vi "OEE_SCREEN_2_worst_ok_count_into_cluster.vi"(6 "SCREEN_2":T1={"header_part_no"="-", "header_customer"="-", "performance_percentage"="-", "performance_target"="-", "performance_actual"="-", "performance_header"="PERFORMANCE", "performance_header_target"="TARGET", "performance_header_actual"="ACTUAL"}, 11 "SCREEN_1":T2={"header_date"="-", "header_time"="-", "header_takt"="-", "header_shift"="-", "OP10_actual"="-", "OP10_rejects"="-", "OP10_quality_yeild"="-", "OP10_pace"="-", "OP20_actual"="-", "OP20_rejects"="-", "OP20_quality_yeild"="-", "OP20_pace"="-", "OP30_actual"="-", "OP30_rejects"="-", "OP30_quality_yeild"="-", "OP30_pace"="-", "OP40_actual"="-", "OP40_rejects"="-", "OP40_quality_yeild"="-", "OP40_pace"="-", "OP50_actual"="-", "OP50_rejects"="-", "OP50_quality_yeild"="-", "OP50_pace"="-", "OP60_actual"="-", "OP60_rejects"="-", "OP60_quality_yeild"="-", "OP60_pace"="-", "OP70_actual"="-", "OP70_rejects"="-", "OP70_quality_yeild"="-", "OP70_pace"="-", "OP80_actual"="-", "OP80_rejects"="-", "OP80_quality_yeild"="-", "OP80_pace"="-", "OP90_actual"="-", "OP90_rejects"="-", "OP90_quality_yeild"="-", "OP90_pace"="-", "OP100_actual"="-", "OP100_rejects"="-", "OP100_quality_yeild"="-", "OP100_pace"="-", "OP110_actual"="-", "OP110_rejects"="-", "OP110_quality_yeild"="-", "OP110_pace"="-", "OP120_actual"="-", "OP120_rejects"="-", "OP120_quality_yeild"="-", "OP120_pace"="-", "OP130_actual"="-", "OP130_rejects"="-", "OP130_quality_yeild"="-", "OP130_pace"="-", "OP10_header"="OP10", "OP20_header"="OP20", "OP30_header"="OP30", "OP40_header"="OP40", "OP50_header"="OP50", "OP60_header"="OP60", "OP70_header"="OP70", "OP80_header"="OP80", "OP90_header"="OP90", "OP100_header"="OP100", "OP110_header"="OP110", "OP120_header"="OP120", "OP130_header"="OP130", "additional_info"="", "bottleneck_OP"="-", "bottleneck_header"="LINE BOTTLENECK"}) -> (4 "SCREEN_2":T1={"header_part_no"="-", "header_customer"="-", "performance_percentage"="-", "performance_target"="-", "performance_actual"="-", "performance_header"="PERFORMANCE", "performance_header_target"="TARGET", "performance_header_actual"="ACTUAL"})   [LabVIEW 2019]
uses:
  <userlib>/_OpenG.lib/array/array.llb/Sort 1D Array (I32)__ogtk.vi
  <userlib>/_OpenG.lib/array/array.llb/Reorder 2D Array2 (String)__ogtk.vi
  SCREEN_1/typedef/SCREEN_1.ctl
  typedef/SCREEN_2.ctl
panel:
  # "Performance Data Output Board #2"
  # "Performance Data Output Board #2"
  # "PERFORMANCE DATA OUTPUT BOARD #1"
  # "OP"
  # "Actual"
  # "Rejects"
  # "%FTTH"
  # "Pace"
  # "OP"
  # "Actual"
  # "Rejects"
  # "%FTTH"
  # "Pace"
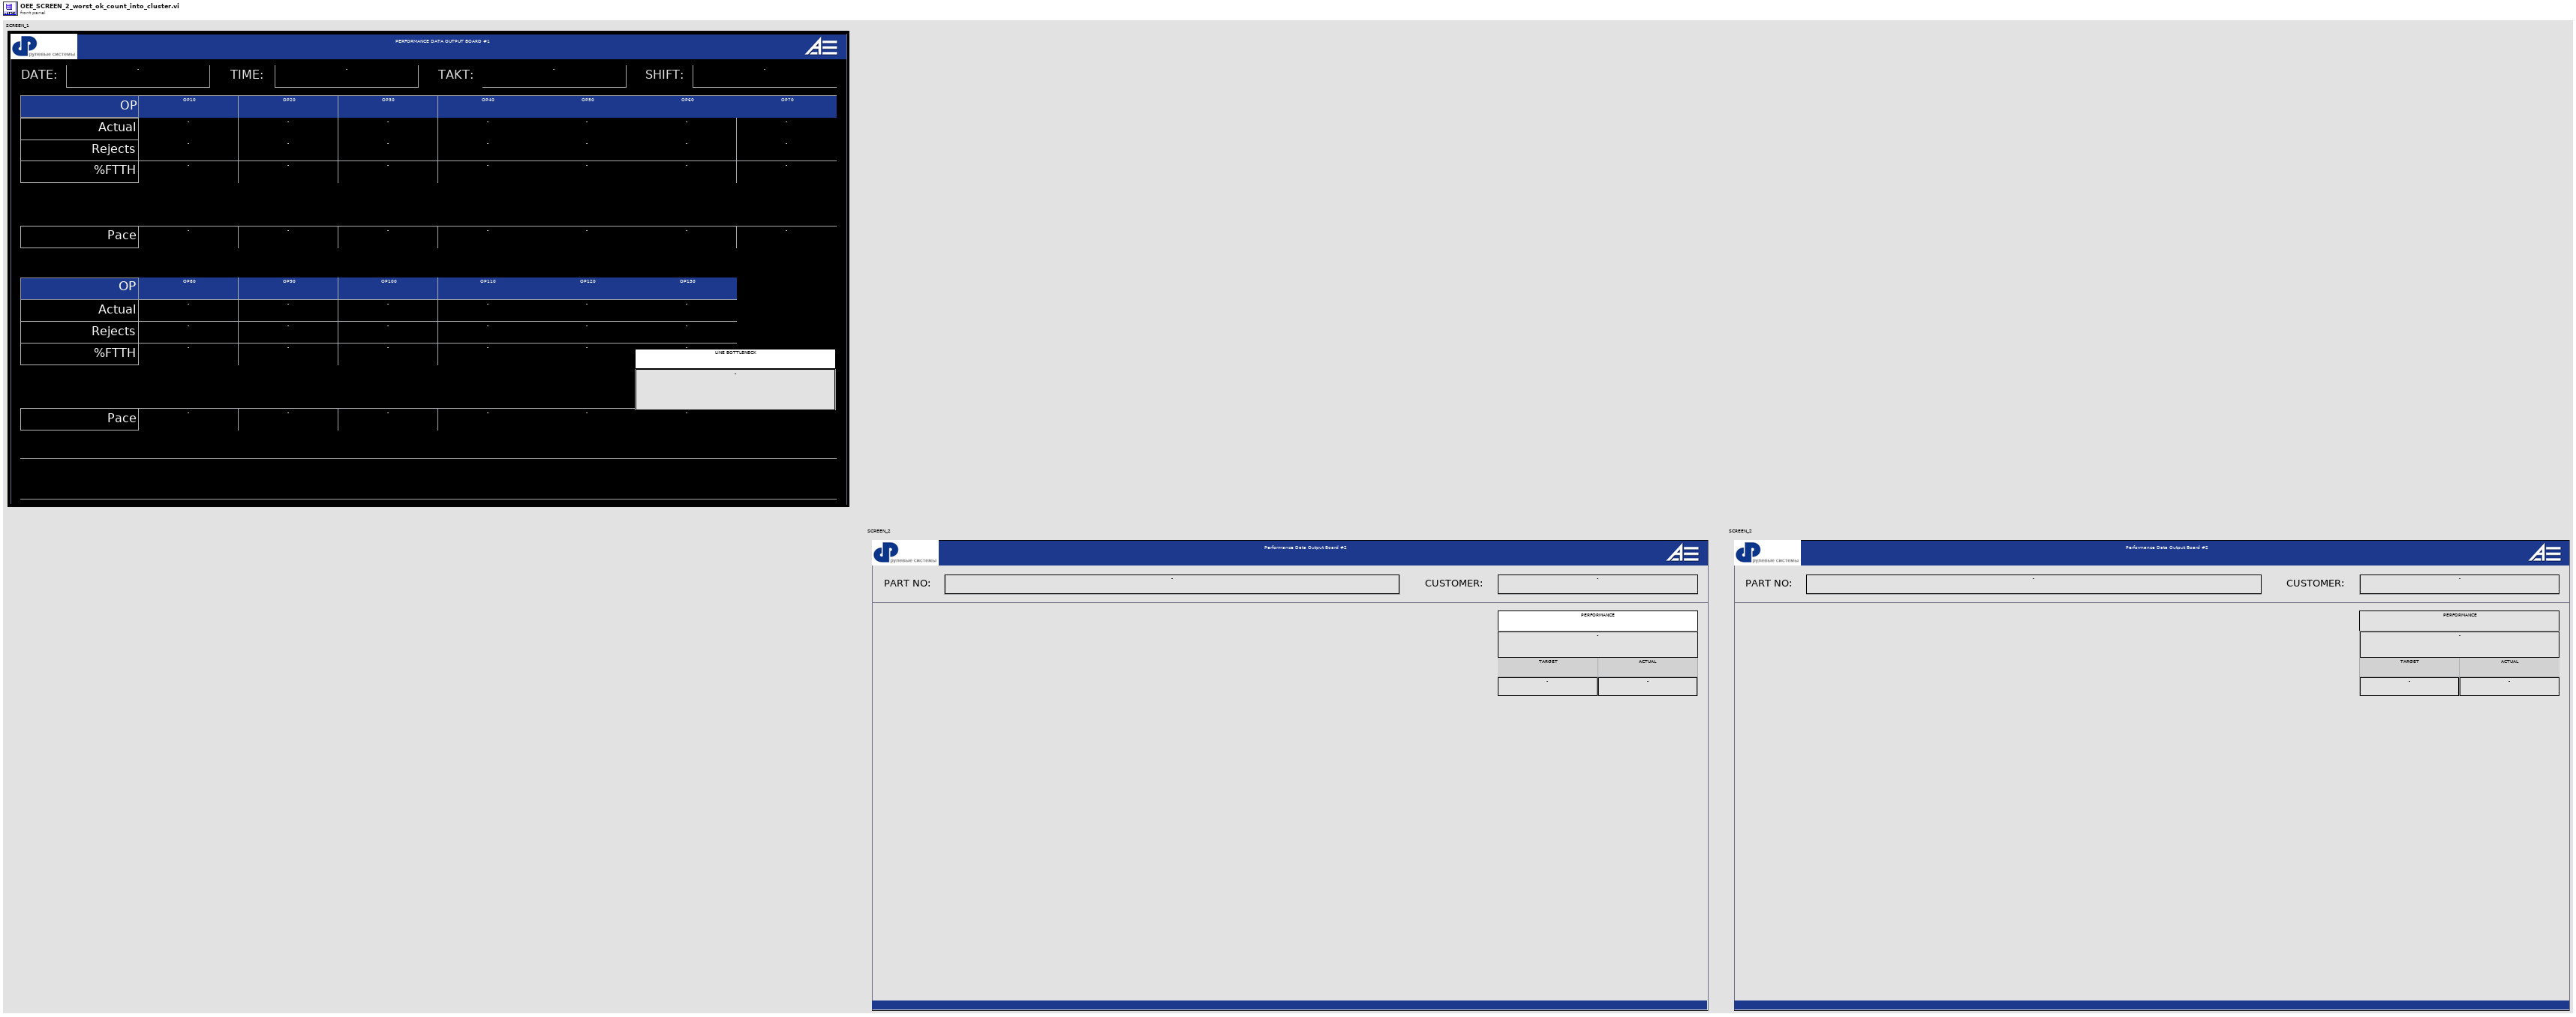
[diagram p1: front panel]
types:
  T1 = typedef "SCREEN_2.ctl" = cluster{"header_part_no":string, "header_customer":string, "performance_percentage":string, "performance_target":string, "performance_actual":string, "performance_header":string, "performance_header_target":string, "performance_header_actual":string}
  T2 = typedef "SCREEN_1.ctl" = cluster{"header_date":string, "header_time":string, "header_takt":string, "header_shift":string, "OP10_actual":string, "OP10_rejects":string, "OP10_quality_yeild":string, "OP10_pace":string, "OP20_actual":string, "OP20_rejects":string, "OP20_quality_yeild":string, "OP20_pace":string, "OP30_actual":string, "OP30_rejects":string, "OP30_quality_yeild":string, "OP30_pace":string, "OP40_actual":string, "OP40_rejects":string, "OP40_quality_yeild":string, "OP40_pace":string, "OP50_actual":string, "OP50_rejects":string, "OP50_quality_yeild":string, "OP50_pace":string, "OP60_actual":string, "OP60_rejects":string, "OP60_quality_yeild":string, "OP60_pace":string, "OP70_actual":string, "OP70_rejects":string, "OP70_quality_yeild":string, "OP70_pace":string, "OP80_actual":string, "OP80_rejects":string, "OP80_quality_yeild":string, "OP80_pace":string, "OP90_actual":string, "OP90_rejects":string, "OP90_quality_yeild":string, "OP90_pace":string, "OP100_actual":string, "OP100_rejects":string, "OP100_quality_yeild":string, "OP100_pace":string, "OP110_actual":string, "OP110_rejects":string, "OP110_quality_yeild":string, "OP110_pace":string, "OP120_actual":string, "OP120_rejects":string, "OP120_quality_yeild":string, "OP120_pace":string, "OP130_actual":string, "OP130_rejects":string, "OP130_quality_yeild":string, "OP130_pace":string, "OP10_header":string, "OP20_header":string, "OP30_header":string, "OP40_header":string, "OP50_header":string, "OP60_header":string, "OP70_header":string, "OP80_header":string, "OP90_header":string, "OP100_header":string, "OP110_header":string, "OP120_header":string, "OP130_header":string, "additional_info":string, "bottleneck_OP":string, "bottleneck_header":string}
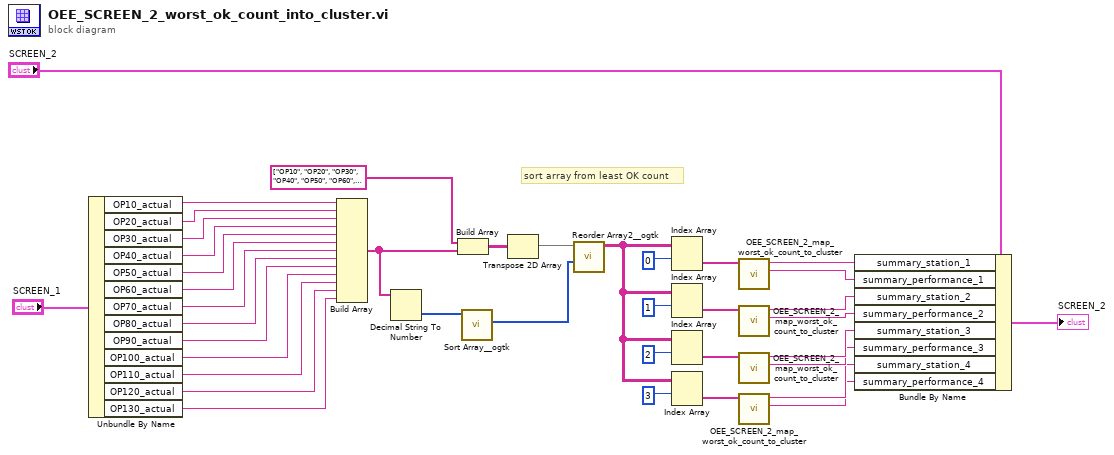
[diagram p0: block diagram]
diagram:
  # "sort array from least OK count"
  n1 = Unbundle By Name("SCREEN_1") -> ("OP10_actual"=w38:string, "OP20_actual"=w37:string, "OP30_actual"=w36:string, "OP40_actual"=w35:string, "OP50_actual"=w34:string, "OP60_actual"=w33:string, "OP70_actual"=w32:string, "OP80_actual"=w31:string, "OP90_actual"=w30:string, "OP100_actual"=w29:string, "OP110_actual"=w28:string, "OP120_actual"=w27:string, "OP130_actual"=w26:string)
  n2 = Build Array(w38, w37, w36, w35, w34, w33, w32, w31, w30, w29, w28, w27, w26) -> (w23:string[])
  n3 = Decimal String To Number(string=w23) -> (number=w25:i32[])  [unwired: 2 in, 1 out]
  n4 = Build Array(string[] ["OP10", "OP20", "OP30", "OP40", "OP50", "OP60", "OP70", "OP80", "OP90", "OP100", "OP110", "OP120", "OP130"], w23) -> (w22:string[][])
  n5 = call-poly <userlib>:"Sort Array__ogtk.vi"("Array in"=w25) -> ("Sorted Pointers"=w20:i32[])  [unwired: 9 in, 1 out]
  n6 = Transpose 2D Array(2D array=w22) -> (transposed array=w21:string[][])
  n7 = call-poly <userlib>:"Reorder Array2__ogtk.vi"("indices"=w20, "array"=w21) -> ("reordered array"=w10:string[][])  [unwired: 9 in]
  n8 = Index Array(array=w10, index (row)=0) -> (element=w13:string[])  [unwired: 1 in]
  n9 = Index Array(array=w10, index (row)=1) -> (element=w9:string[])  [unwired: 1 in]
  n10 = Index Array(array=w10, index (row)=2) -> (element=w8:string[])  [unwired: 1 in]
  n11 = Index Array(array=w10, index (row)=3) -> (element=w7:string[])  [unwired: 1 in]
  n12 = call "OEE_SCREEN_2_map_worst_ok_count_to_cluster.vi"("worst_ok_record"=w13) -> ("performance"=w11:string, "station"=w12:string)  [unwired: 9 in]
  n13 = call "OEE_SCREEN_2_map_worst_ok_count_to_cluster.vi"("worst_ok_record"=w9) -> ("performance"=w5:string, "station"=w6:string)  [unwired: 9 in]
  n14 = call "OEE_SCREEN_2_map_worst_ok_count_to_cluster.vi"("worst_ok_record"=w8) -> ("performance"=w3:string, "station"=w4:string)  [unwired: 9 in]
  n15 = call "OEE_SCREEN_2_map_worst_ok_count_to_cluster.vi"("worst_ok_record"=w7) -> ("performance"=w1:string, "station"=w2:string)  [unwired: 9 in]
  n16 = Bundle By Name(cluster="SCREEN_2", "summary_station_1"=w12, "summary_performance_1"=w11, "summary_station_2"=w6, "summary_performance_2"=w5, "summary_station_3"=w4, "summary_performance_3"=w3, "summary_station_4"=w2, "summary_performance_4"=w1) -> (→"SCREEN_2":T1)
